vi "Reject Wrong Cargo (SubVI).vi"(6 "cargoSensors":T1, 9 "desiredIntakePosition":dbl, 10 "desiredIndexerOutput":dbl, 11 "desiredIntakeOutput":dbl) -> (1 "desiredIntakePosition":dbl, 2 "desiredIndexerOutput":dbl, 3 "desiredIntakeOutput":dbl)   [LabVIEW 2020]
uses:
  <vilib>/Rock Robotics/WPI/ThirdParty/JAS_Junk/TrajLib/Trajectory_Library.lvlib
  Cargo Sensors.ctl
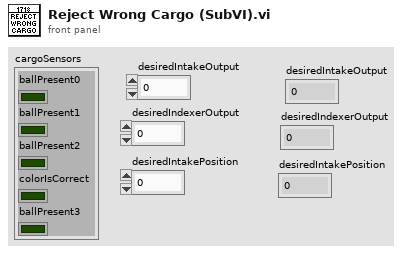
[diagram p1: front panel]
types:
  T1 = typedef "Cargo Sensors.ctl" = cluster{"ballPresent0":bool, "ballPresent1":bool, "ballPresent2":bool, "colorIsCorrect":bool, "ballPresent3":bool}
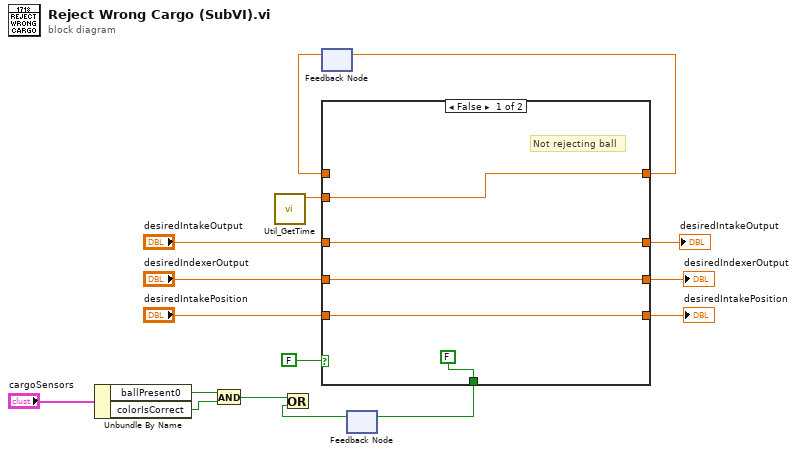
[diagram p0: block diagram]
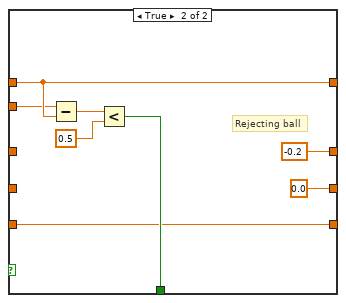
[diagram p2: hidden frame]
diagram:
  n1 = Unbundle By Name("cargoSensors") -> ("ballPresent0"=w9:bool, "colorIsCorrect"=w10:bool)
  n2 = And(x=w9, y=w10) -> (x .and. y?=w11:bool)
  n3 = call <vilib>:"Util_GetTime.vi"() -> ("FPGA_Time_Seconds"=w1:dbl)  [unwired: 10 in, 1 out]
  n4 = feedback #1() -> (w3:dbl)  [unwired: 1 in]
  n5 = case shown="False" FALSE {
    tunnel: "desiredIntakeOutput" -> [w21 _]
    tunnel: "desiredIndexerOutput" -> [w20 _]
    tunnel: [w21 -0.2 ("Intake")] -> w7
    tunnel: [w20 0.0 ("Intake")] -> w8
    tunnel: w1 -> [w19 w26]
    tunnel: [w19 w27] -> w2
    tunnel: w3 -> [_ w27]
    tunnel: [FALSE w23] -> w4
    tunnel: "desiredIntakePosition" -> [w17 w22]
    tunnel: [w17 w22] -> w13
    frame False {
      # "Not rejecting ball"
    }
    frame True {
      # "Rejecting ball"
      n6 = Subtract(x=w26, y=w27) -> (x-y=w25:dbl)
      n7 = Less?(x=w25, y=0.5) -> (x < y?=w23:bool)
    }
  }
  "desiredIntakePosition" <- w13
  "desiredIndexerOutput" <- w8
  "desiredIntakeOutput" <- w7
  n8 = feedback-in #1(w2) -> ()
  n9 = feedback #2() -> (w5:bool)  [unwired: 1 in]
  n10 = Or(x=w11, y=w5) -> ()  [unwired: 1 out]
  n11 = feedback-in #2(w4) -> ()
